vi "WLAN_BCCDecode.vi"(8 "error in (no error)":errorcluster, 9 "need add zeros?":bool, 10 "BCC rate (k/n)":enum16{"1/2", "2/3", "3/4"}(ring), 11 "input bit stream":i8[](array[numeric])) -> (0 "error out":errorcluster, 3 "output bit stream":i8[](array[numeric]))   [LabVIEW 2014]
uses:
  <vilib>/addons/Modulation/Digital/Channel Coding/MT Convolutional Decoder (Viterbi Hard Decision, Generator Matrix).vi
  <vilib>/addons/Modulation/niDMT.lvlib
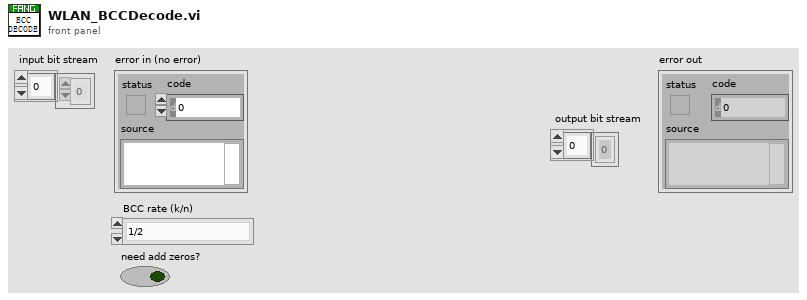
[diagram p1: front panel]
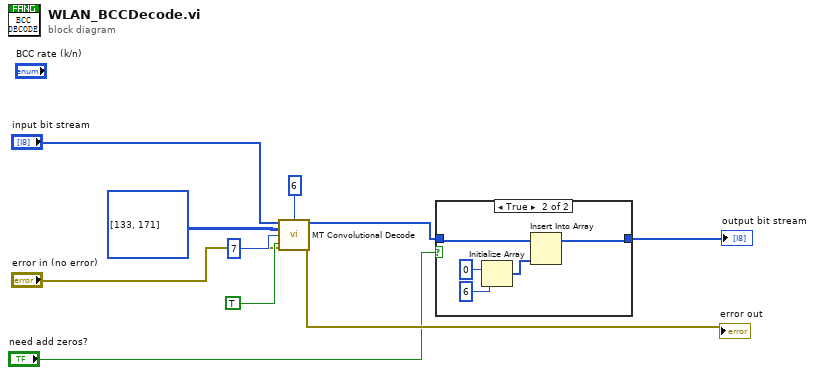
[diagram p0: block diagram]
diagram:
  n1 = call-poly <vilib>:"MT Convolutional Decode.vi"("input bit stream"="input bit stream", "traceback depth (D)"=6, "generator matrix (n x k)"=u32[][] [[133], [171]], "constraint length (K)"=7, "error in (no error)"="error in (no error)", "reset? (T)"=TRUE) -> ("output bit stream"=w1:i8[], "error out"=→"error out":errorcluster)  [unwired: 7 in, 1 out]
  n2 = case shown="True" "need add zeros?" {
    tunnel: [w11 w12] -> w2
    tunnel: w1 -> [w11 w16]
    frame False {
    }
    frame True {
      n3 = Initialize Array(i8 0 ("element"), 6 ("dimension size")) -> (w15:i8[])
      n4 = Insert Into Array(array=w16, new element=w15) -> (w12:i8[])  [unwired: 1 in]
    }
  }
  "output bit stream" <- w2
